vi "Replace empty string with NULL.vi"(11 "String in":string) -> (3 "string out":string)   [LabVIEW 2020]
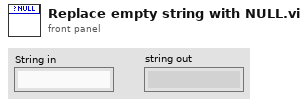
[diagram p1: front panel]
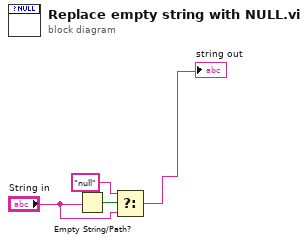
[diagram p0: block diagram]
diagram:
  n1 = Empty String/Path?(string/path="String in") -> (empty?=w1:bool)
  n2 = Select(t="null", s=w1, f="String in") -> (s? t:f=→"string out":string)
